vi "RightHaveSameStone.vi"(0 "Row in":i32, 1 "StoneColor":u16, 5 "Col in":i32, 7 "Chessboard":T1, 9 "TatgetIndex":T2, 11 "error in (no error)":errorcluster) -> (3 "HaveSameStone?":bool, 4 "Row out":i32, 6 "Col out":i32, 8 "Chessboard out":T1, 10 "SSIndex":T2, 15 "error out":errorcluster)   [LabVIEW 2009]
doc: "To seek same stone in the Right direction.\n--------------------------------------------\nStoneColor: Witch stone type is seeking for.\nRow in: Start index number(Row).\nCol in: Start index number(Col).\nChessboard: The Chessboard seeking on.\nTargetIndex: Index mumber the seeking ends.\nHaveSameStone: If there are same stones this indicator returns TRUE.\nRow out: Pass out the start index number(Row).\nCol out: Pass out the start index number(Col).\nChessboard out: Pass out the Chessboard seeking on.\nSSIndex: Return the Index numbers of same stone."
uses:
  Controls/Chess.ctl
  Controls/ItemIndex.ctl
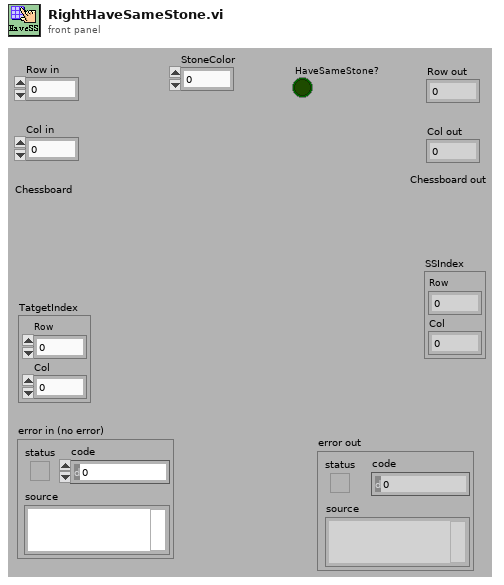
[diagram p1: front panel]
types:
  T1 = typedef "Chess.ctl" = u16[][]
  T2 = typedef "ItemIndex.ctl" = cluster{"Row":i32, "Col":i32}
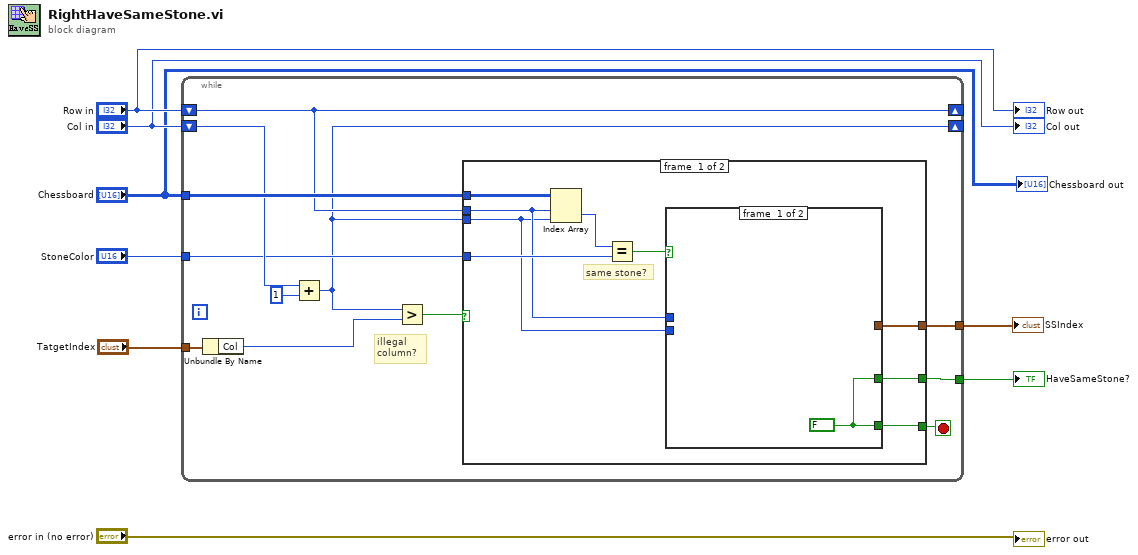
[diagram p0: block diagram]
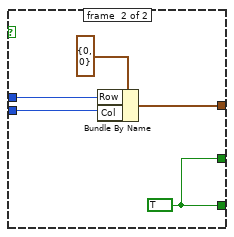
[diagram p2: hidden frame]
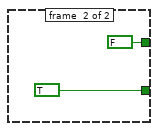
[diagram p3: hidden frame]
diagram:
  n1 = while {
    tunnel: "Chessboard" -> [w19]
    tunnel: "StoneColor" -> [w16]
    shift-right: [w17] -> _
    shift-left: "Row in" -> [w17]
    shift-right: [w11] -> _
    shift-left: "Col in" -> [w18]
    tunnel: [w15] -> w8
    tunnel: [w14] -> w5
    tunnel: "TatgetIndex" -> [w13]
    stop <- w20 stop-if-true
    # "illegal \ncolumn?"
    n2 = Unbundle By Name(w13) -> ("Col"=w10:i32)
    n3 = Add(x=w18, y=1) -> (x+y=w11:i32)
    n4 = Greater?(x=w11, y=w10) -> (0:w12:bool)
    n5 = case shown="True" w12 {
      tunnel: [w26 TRUE] -> w20
      tunnel: w19 -> [w29 _]
      tunnel: w11 -> [w22 _]
      tunnel: w17 -> [w23 _]
      tunnel: w16 -> [w25 _]
      tunnel: [w24 FALSE] -> w15
      tunnel: [w21 _] -> w14
      frame #0 {
        # "same stone?"
        n6 = Index Array(array=w29, index (row)=w23, index (col)=w22) -> (element=w28:u16)
        n7 = Equal?(x=w28, y=w25) -> (x = y?=w27:bool)
        n8 = case shown="False" w27 {
          tunnel: [w30 w35] -> w26
          tunnel: [w30 w35] -> w24
          tunnel: w23 -> [_ w33]
          tunnel: w22 -> [_ w32]
          tunnel: [_ w31] -> w21
          frame #0 {
            w30 = FALSE
          }
          frame #1 {
            w35 = TRUE
            n9 = Bundle By Name(cluster=T2 {"Row"=0, "Col"=0} ("ItemIndex"), "Row"=w33, "Col"=w32) -> (w31:T2)
          }
        }
      }
      frame #1 {
      }
    }
  }
  "HaveSameStone?" <- w8
  "SSIndex" <- w5
  "Col out" <- "Col in"
  "Row out" <- "Row in"
  "error out" <- "error in (no error)"
  "Chessboard out" <- "Chessboard"
